vi "Reply.vi"(8 "error in (no error)":errorcluster, 11 "Self-addressed Msg in":refnum<class "Self-addressed Msg.lvclass">) -> (0 "error out":errorcluster, 3 "Self-addressed Msg out":refnum<class "Self-addressed Msg.lvclass">)   [LabVIEW 2015, in "Self-addressed Msg.lvclass"]
uses:
  Self-addressed Msg.lvclass
  Self-addressed Msg.lvclass/Self-addressed Msg.ctl
  <vilib>/ActorFramework/Message Enqueuer/Message Enqueuer.lvclass/Message Enqueuer.ctl
  <vilib>/ActorFramework/Message Priority Queue/Priority Enqueue.vi
  <vilib>/ActorFramework/Message Enqueuer/Message Enqueuer.lvclass
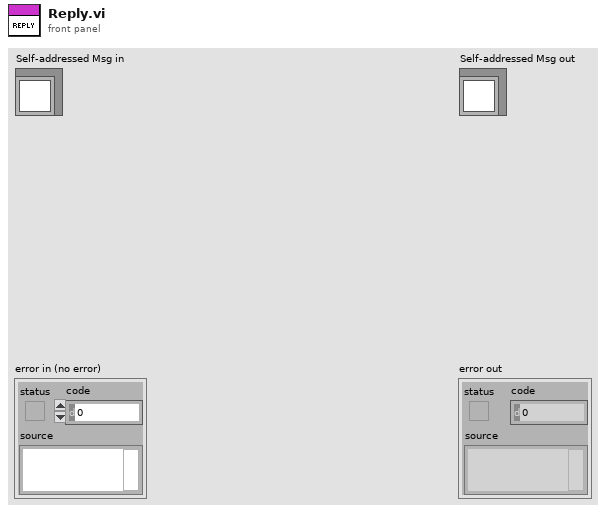
[diagram p1: front panel]
types:
  T1 = typedef "Actor Framework.lvlib/Message Enqueuer.lvclass/Message Priority.ctl" = enum16{"Low", "Normal", "High"}
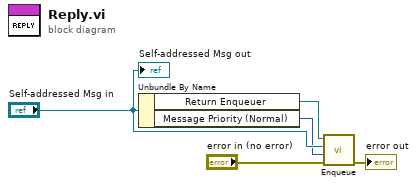
[diagram p0: block diagram]
diagram:
  n1 = Unbundle By Name("Self-addressed Msg in") -> ("Return Enqueuer"=w4:refnum<class "Message Enqueuer.lvclass">, "Message Priority (Normal)"=w1:T1)
  n2 = call <vilib>:"Enqueue.vi"("error in (no error)"="error in (no error)", "Message Priority (Normal)"=w1, "Message"="Self-addressed Msg in", "Message Enqueuer in"=w4) -> ("error out"=→"error out":errorcluster)  [unwired: 6 in, 1 out]
  "Self-addressed Msg out" <- "Self-addressed Msg in"
